vi "Receive Signal.vi"(8 "error in":errorcluster, 10 "Frame.Signal":string, 11 "ICommunicate in":refnum<class "ICAN.lvclass">) -> (0 "error out":errorcluster, 2 "Value":dbl, 3 "ICommunicate out":refnum<class "ICAN.lvclass">)   [LabVIEW 2023, in "ICAN.lvclass"]
uses:
  ICAN.lvclass
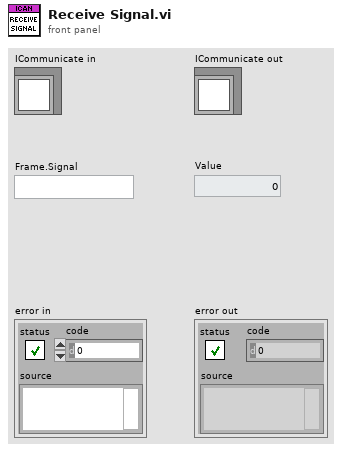
[diagram p1: front panel]
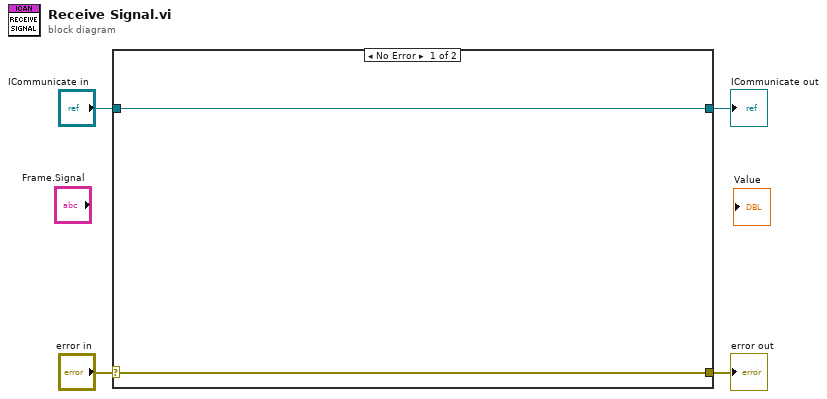
[diagram p0: block diagram]
diagram:
  n1 = case shown="No Error" "error in" {
    selector: "error in" -> [w5 w8]
    tunnel: [w5 w8] -> w3
    tunnel: [w6 w7] -> w1
    tunnel: "ICommunicate in" -> [w6 w7]
    frame No Error {
    }
    frame Error {
    }
  }
  "error out" <- w3
  "ICommunicate out" <- w1
